vi "Build Maps Pair Array.vi"(11 "Keypad":string[][](array[string])) -> (1 "Pos-Key Map Out":map{T2, string}(c390), 2 "Key-Pos Map Out":map{string, T2}(c390), 3 "Pair Array Out":T1[](array[typedef]), 5 "Button Array Out":string[](array[string]))   [LabVIEW 2024]
uses:
  Utility/Universal Utility/TypeDefs_Utility/Cluster_Row-Column.ctl
  Cluster_Start-End Keys.ctl
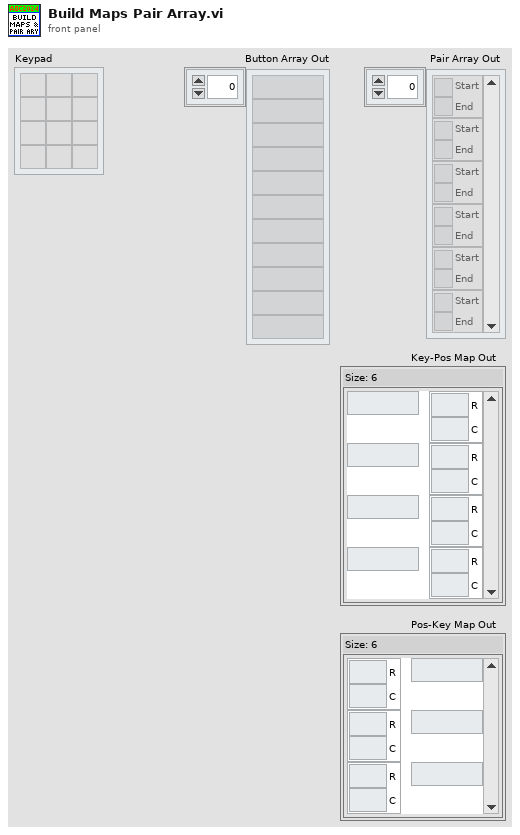
[diagram p1: front panel]
types:
  T1 = typedef "Cluster_Start-End Keys.ctl" = cluster{"Start":string, "End":string}
  T2 = typedef "Cluster_Row-Column.ctl" = cluster{"R":i32, "C":i32}
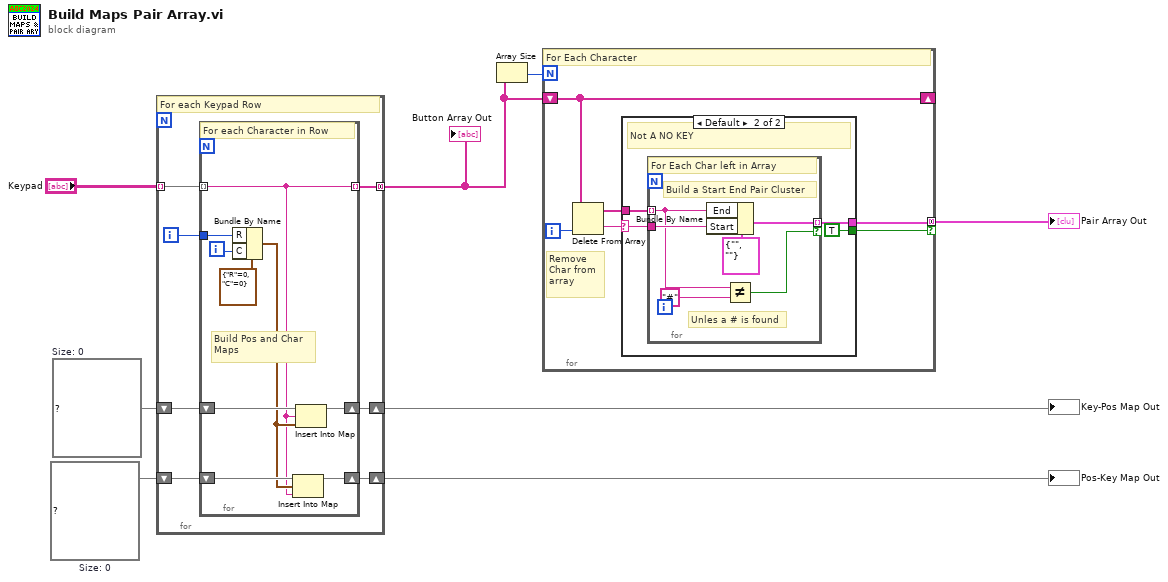
[diagram p0: block diagram]
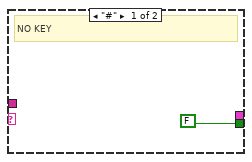
[diagram p2: hidden frame]
diagram:
  w4 = map{T2, string} {}  # Size: 0
  w3 = map{string, T2} {}  # Size: 0
  n1 = for {
    tunnel: "Keypad" -> [w15] mode=indexing
    tunnel: [w13] -> w1 mode=concatenating
    shift-right: [w11] -> w6
    shift-left: w3 -> [w12]
    shift-right: [w9] -> w7
    shift-left: w4 -> [w10]
    i -> [w14]
    # "For each Keypad Row"
    n2 = for {
      tunnel: w15 -> [w16] mode=indexing
      tunnel: w14 -> [w23]
      tunnel: [w16] -> w13 mode=indexing
      shift-right: [w20] -> w11
      shift-left: w12 -> [w21]
      shift-right: [w18] -> w9
      shift-left: w10 -> [w19]
      i -> [w22]
      # "Build Pos and Char\nMaps"
      # "For each Character in Row"
      n3 = Bundle By Name(cluster=T2 {"R"=0, "C"=0} ("Position"), "R"=w23, "C"=w22) -> (w17:T2)
      n4 = Insert Into Map(map in=w19, key=w17, value=w16) -> (map out=w18:map{T2, string})  [unwired: 2 out]
      n5 = Insert Into Map(map in=w21, key=w16, value=w17) -> (map out=w20:map{string, T2})  [unwired: 2 out]
    }
  }
  "Button Array Out" <- w1
  "Pos-Key Map Out" <- w7
  "Key-Pos Map Out" <- w6
  n6 = Array Size(array=w1) -> (size(s)=w2:i32)
  n7 = for {
    N: w2 -> [_]
    shift-right: [w27] -> _
    shift-left: w1 -> [w27]
    tunnel: [w28] -> w5 mode=concatenating if=w25
    i -> [w29]
    # "Remove\nChar from\narray"
    # "For Each Character"
    n8 = Delete From Array(array=w27, index=w29) -> (deleted portion=w30:string, array with subset deleted=w26:string[])  [unwired: 1 in]
    n9 = case shown="Default" w30 {
      selector: w30 -> [_ w35]
      tunnel: [_ w34] -> w28
      tunnel: w26 -> [_ w33]
      tunnel: [FALSE TRUE] -> w25
      frame "#" {
        # "NO KEY"
      }
      frame Default {
        # "Not A NO KEY"
        n10 = for {
          tunnel: w35 -> [w38]
          tunnel: w33 -> [w37] mode=indexing
          tunnel: [w41] -> w34 mode=indexing if=w36
          # "Unles a # is found"
          # "Build a Start End Pair Cluster"
          # "For Each Char left in Array"
          n11 = Bundle By Name(cluster=T1 {"Start"="", "End"=""} ("output cluster"), "End"=w37, "Start"=w38) -> (w41:T1)
          n12 = Not Equal?(x=w37, y="#") -> (x != y?=w36:bool)
        }
      }
    }
  }
  "Pair Array Out" <- w5
